vi "Remove scrollbars.vi"(8 "error in (no error)":errorcluster, 11 "VI in":refnum<vi>) -> (0 "error out":errorcluster)   [LabVIEW 2026, in "TALOS.lvlib" / "Common GUI v3.lvlib" / "Common GUI v3.lvclass"]
uses:
  Common GUI v3.lvclass
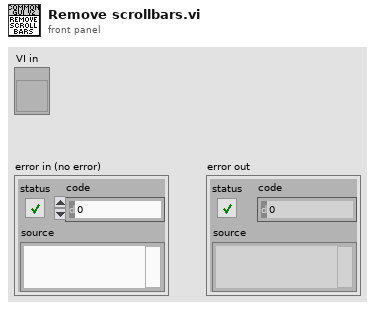
[diagram p1: front panel]
types:
  T1 = enum16{"Always On", "Always Off", "Off While Running"}
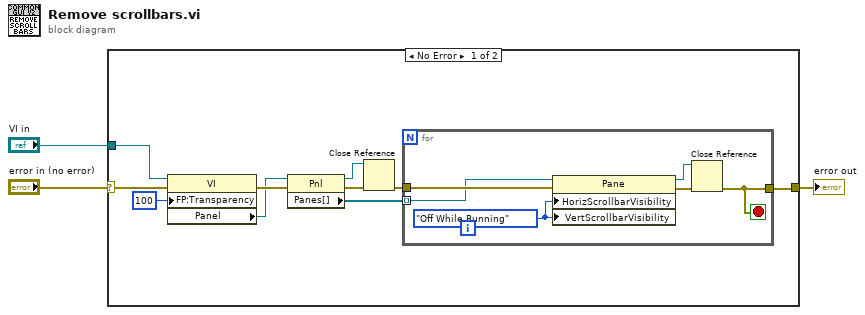
[diagram p0: block diagram]
diagram:
  n1 = case shown="No Error" "error in (no error)" {
    selector: "error in (no error)" -> [w11 w20]
    tunnel: [w7 w20] -> w3
    tunnel: "VI in" -> [w10 _]
    frame No Error {
      n2 = property class="VI"(reference=w10, error in=w11, "FP:Transparency"=u8 100 ("Front Panel Window:Transparency")) -> (error out=w12:errorcluster, "Panel"=w5:refnum<vi>)  [unwired: 1 out]
      n3 = property class="Pnl"(reference=w5, error in=w12) -> (reference out=w6:refnum<vi>, error out=w13:errorcluster, "Panes[]"=w8:refnum<vi>[])
      n4 = Close Reference(reference=w6, error in (no error)=w13) -> (error out=w9:errorcluster)
      n5 = for {
        tunnel: w9 -> [w19]
        tunnel: w8 -> [w18] mode=indexing
        tunnel: [w14] -> w7
        stop <- w14 stop-if-true
        w17 = T1."Off While Running" ("Vertical Scrollbar Visibility")
        n6 = property class="Pane"(reference=w18, error in=w19, "HorizScrollbarVisibility"=w17, "VertScrollbarVisibility"=w17) -> (reference out=w15:refnum<vi>, error out=w16:errorcluster)
        n7 = Close Reference(reference=w15, error in (no error)=w16) -> (error out=w14:errorcluster)
      }
    }
    frame Error {
    }
  }
  "error out" <- w3
